vi "Sort Sequence List.vi"(1 "Sequence Data In":T1[](array[typedef])) -> (0 "Sequence Data Out":T1[](array[typedef]))   [LabVIEW 2020]
uses:
  Control/Setup - Sequence Data.ctl
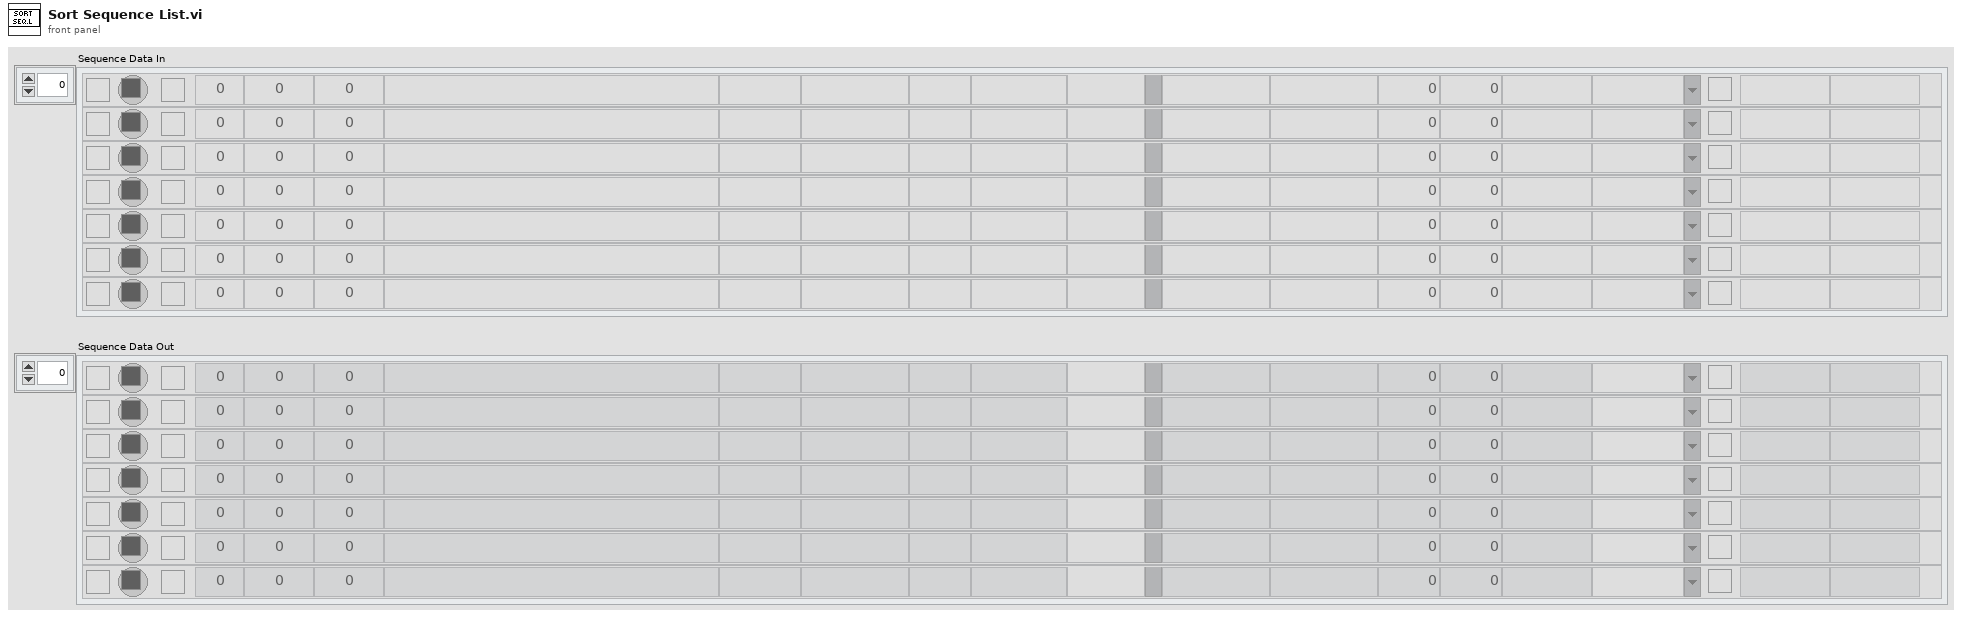
[diagram p1: front panel]
types:
  T1 = typedef "Setup - Sequence Data.ctl" = cluster{"Seq.Select":bool, "Seq.Status":u32, "Seq.Run":bool, "Seq.TestSequence":dbl, "Seq.No":dbl, "Seq.ReqID":string, "Seq.TestReq":string, "Seq.Variance":string, "Seq.TestProcedure":string, "Seq.Section":string, "Seq.TestSystem":string, "Seq.TestPressure":string, "Seq.Cycle":string, "Seq.TestGroup":dbl, "Seq.MSHP":dbl, "Seq.PHPD":dbl, "Seq.HoldingTime":string, "Seq.ChartScale":string, "Seq.ActuatorPressure":string, "Seq.MaxBDPressure":string, "Seq.BDIndicator":bool, "Seq.TestMedia":string}
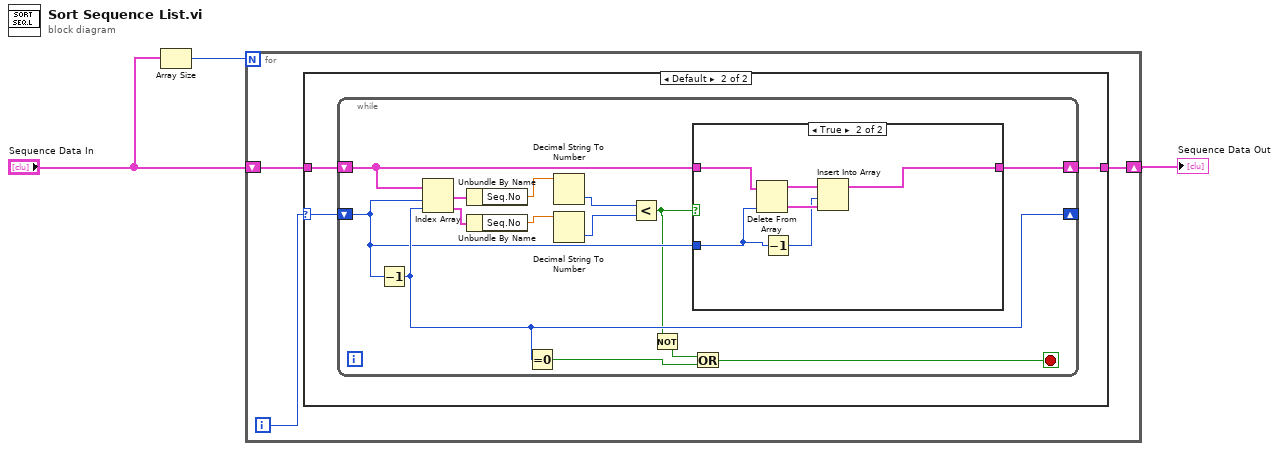
[diagram p0: block diagram]
diagram:
  n1 = Array Size(array="Sequence Data In") -> (size(s)=w2:i32)
  n2 = for {
    N: w2 -> [_]
    shift-right: [w4] -> w1
    shift-left: "Sequence Data In" -> [w5]
    i -> [w6]
    n3 = case shown="Default" w6 {
      selector: w6 -> [_ w9]
      tunnel: w5 -> [w7 w10]
      tunnel: [w7 w8] -> w4
      frame 0 {
      }
      frame Default {
        n4 = while {
          shift-right: [w21] -> _
          shift-left: w9 -> [w20]
          shift-right: [w19] -> w8
          shift-left: w10 -> [w22]
          stop <- w17 stop-if-true
          n5 = Decrement(x=w20) -> (x-1=w21:i32)
          n6 = Index Array(array=w22, index #1=w20, index #2=w21) -> (element #1=w24:T1, element #2=w23:T1)
          n7 = Unbundle By Name(w24) -> ("Seq.No"=w14:dbl)
          n8 = Unbundle By Name(w23) -> ("Seq.No"=w13:dbl)
          n9 = Equal To 0?(x=w21) -> (x = 0?=w18:bool)
          n10 = Decimal String To Number(string=w14) -> (number=w12:i32)  [unwired: 2 in, 1 out]
          n11 = Decimal String To Number(string=w13) -> (number=w11:i32)  [unwired: 2 in, 1 out]
          n12 = Less?(x=w12, y=w11) -> (x < y?=w16:bool)
          n13 = Not(x=w16) -> (.not. x?=w15:bool)
          n14 = case shown="True" w16 {
            tunnel: w22 -> [w25 w31]
            tunnel: w20 -> [_ w28]
            tunnel: [w25 w26] -> w19
            frame False {
            }
            frame True {
              n15 = Delete From Array(array=w31, index=w28) -> (deleted portion=w29:T1, array with subset deleted=w30:T1[])  [unwired: 1 in]
              n16 = Decrement(x=w28) -> (x-1=w27:i32)
              n17 = Insert Into Array(array=w30, index=w27, new element=w29) -> (w26:T1[])
            }
          }
          n18 = Or(x=w15, y=w18) -> (x .or. y?=w17:bool)
        }
      }
    }
  }
  "Sequence Data Out" <- w1
